vi "Read Results.lvclass.vi"(8 "error in (no error)":errorcluster, 11 "Display Results in":refnum<class "Display Results.lvclass">) -> (0 "error out":errorcluster, 2 "Results.lvclass":refnum<class "Results.lvclass">, 3 "Display Results out":refnum<class "Display Results.lvclass">)   [LabVIEW 2017, in "Measurement UI.lvlib" / "Display Results.lvclass"]
uses:
  Display Results.lvclass
  Results/Results.lvclass
  Display Results.lvclass/Display Results.ctl
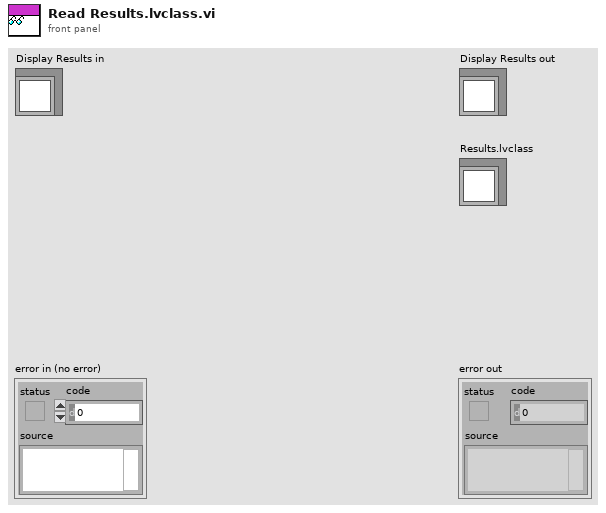
[diagram p1: front panel]
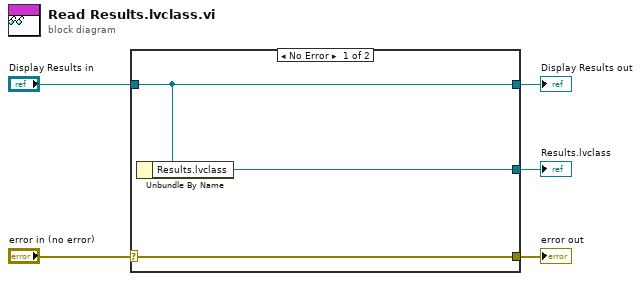
[diagram p0: block diagram]
diagram:
  n1 = case shown="No Error" "error in (no error)" {
    selector: "error in (no error)" -> [w8 w9]
    tunnel: [w8 w9] -> w4
    tunnel: [w7 w10] -> w2
    tunnel: "Display Results in" -> [w7 w10]
    tunnel: [w6 _] -> w1
    frame No Error {
      n2 = Unbundle By Name(w7) -> ("Results.lvclass"=w6:refnum<class "Results.lvclass">)
    }
    frame Error {
    }
  }
  "error out" <- w4
  "Display Results out" <- w2
  "Results.lvclass" <- w1
